vi "DRC.vi"(0 "System no.":i32=1 min=1 max=4 step=1, 2 "Rec. table":i32, 3 "Rec. option":i32, 5 "error in":errorcluster, 6 "Source ID":string, 7 "Trigger option":i32) -> (14 "Controller error":bool, 19 "error out":errorcluster)   [LabVIEW 2020]
doc: "This VI configures the data recording, waits 100 ms and queries ERR?. See GCS DLL manual or user manual for available recording and trigger options. \nGCS 2.0: Trigger option must be 0.\nController error is TRUE if selected system reports an error code which is not 0. \n\nC-843: Trigger option must be 0. See user manual for available record options. The C-843 has four data recorder tables. The available points per table depend on the host computer's memory only. Some hardware revisions do not allow the parallel use of DIO and the data recorder. To switch between both, the C-843 needs to be reconnected.\n\nC-866: Trigger option must be 0. See C-866_GCS_Commands_SM150E.pdf for available record options.\n\nC-867: See user manual for available record options.The C-867 has four data recorder tables with 8192 points per table.\n\nC-877: See user manual for available record options, number of data recorder tables and points per table. Trigger option must be 0.\n\nC-884: See user manual for available record options. Trigger option must be 0. The C-884 has eight data recorder tables with 8192 points per table. \n\nC-891: See user manual for available record options.Trigger option must be 0. The C-891 has four data recorder tables with 4096 points per table. The number of tablescan be changed to 1, 2 or 8 by setting the appropriate parameter value, see User Manual for details.\n\nE-517, E-518: Trigger option must be 0. See user manual for available record options. The number of data recorder tables is 3 with 8192 points per table. The current data recorder configuration is saved with WPA, in addition to the current parameter values and other settings.\n\nE-709: See user manual for available record options. Trigger option must be 0. By default, the number of data recorder tables is 4. It can be reduced by setting the appropriate parameter value, see user manual for details.\n\nE-710: Rec. table and Source ID must be identical.\n\nC-413, E-712, E-725,E-727,E-753, E-754: Trigger option must be 0. See user manual for available record options. By default, the number of data recorder tables is 8. It can be reduced by setting the appropriate parameter value, see user manual for details.\n\nE-861: Trigger option must be 0. See user manual for available record options. The E-861 has two data recorder tables with 1024 points per table.\n\nE-871, E-873: Trigger option must be 0. See user manual for available record options. The E-871, E-873 has two data recorder tables with 1024 points per table. \n\nE-874: Trigger option must be 0. See user manual for available record options. The E-874 has two data recorder tables with 1024 points per table. \n\nC-887, F-206, M-8X0: Only for GCS syntax version = GCS 2.0 or higher (Check with CSV?.vi. If CSV?.vi is not supported, syntax version is GCS 1.0). See user manual for available record options, trigger options, number of data recorder tables and points per table. The number of points can be changed by setting the appropriate parameter value, see user manual of the controller for details.\n\nMercury_GCS: Trigger option must be 0. See user manual for available record options, number of data recorder tables and points per table."
panel:
  # "This vi configures the data recording, waits 100 ms and queries ERR?. \nSee GCS DLL manual or User manual for available recording and trigger \noptions."
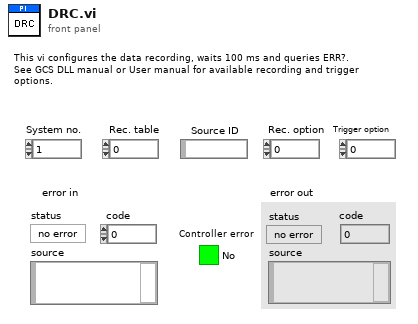
[diagram p1: front panel]
types:
  T1 = enum16{"Disable error check", "Force error check", "Use global settings"}
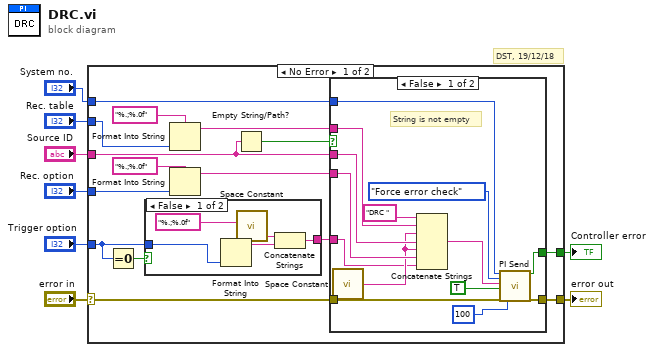
[diagram p0: block diagram]
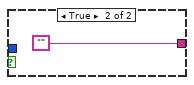
[diagram p2: hidden frame]
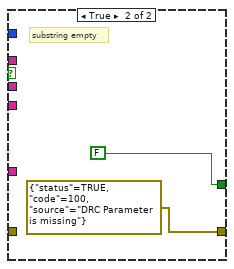
[diagram p3: hidden frame]
diagram:
  # "DST, 19/12/18"
  n1 = case shown="No Error" "error in" {
    selector: "error in" -> [w11 w46]
    tunnel: [w23 w46] -> w8
    tunnel: "System no." -> [w22 _]
    tunnel: "Rec. table" -> [w19 _]
    tunnel: "Rec. option" -> [w18 _]
    tunnel: "Source ID" -> [w10 _]
    tunnel: "Trigger option" -> [w13 _]
    tunnel: [w12 FALSE ("Controller error")] -> w2
    frame No Error {
      n2 = Equal To 0?(x=w13) -> (x = 0?=w15:bool)
      n3 = case shown="False" w15 {
        tunnel: [w24 ""] -> w14
        tunnel: w13 -> [w27 _]
        frame False {
          n4 = Format Into String(format string="%.;%.0f" ("Format String"), w27) -> (resulting string=w26:string)  [unwired: 2 in, 1 out]
          n5 = call "Space Constant.vi"() -> ("String"=w25:string)
          n6 = Concatenate Strings(w25, w26) -> (w24:string)
        }
        frame True {
        }
      }
      n7 = Format Into String(format string="%.;%.0f" ("Format String"), w19) -> (resulting string=w17:string)  [unwired: 2 in, 1 out]
      n8 = Format Into String(format string="%.;%.0f" ("Format String"), w18) -> (resulting string=w16:string)  [unwired: 2 in, 1 out]
      n9 = Empty String/Path?(string/path=w10) -> (empty?=w9:bool)
      n10 = case shown="False" w9 {
        tunnel: [w31 errorcluster {"status"=TRUE, "code"=100, "source"="DRC Parameter is missing"} ("error out")] -> w23
        tunnel: w11 -> [w40 _]
        tunnel: w22 -> [w39 _]
        tunnel: w17 -> [w38 _]
        tunnel: w10 -> [w37 _]
        tunnel: w16 -> [w36 _]
        tunnel: w14 -> [w34 _]
        tunnel: [w30 FALSE ("Controller error")] -> w12
        frame False {
          # "String is not empty"
          n11 = call "Space Constant.vi"() -> ("String"=w35:string)
          n12 = Concatenate Strings("DRC ", w38, w35, w37, w35, w36, w34) -> (w41:string)
          n13 = call "PI Send.vi"("System no."=w39, "Error check settings"=T1."Force error check", "String to send"=w41, "Attach termination char.?"=TRUE ("Attach Linefeed?"), "error in"=w40, "Delay before error check (ms)"=u32 100 ("milliseconds to wait")) -> ("Controller error"=w30:bool, "error out"=w31:errorcluster)  [unwired: 12 out]
        }
        frame True {
          # "substring empty"
        }
      }
    }
    frame Error {
    }
  }
  "error out" <- w8
  "Controller error" <- w2
